vi "Is Call Cancelled.vi"(8 "error in (no error)":errorcluster, 11 "gRPCid in":T1) -> (0 "error out":errorcluster, 2 "Is Cancelled":bool, 3 "gRPCid":T1)   [LabVIEW 2019, in "gprc-lvsupport.lvlib"]
uses:
  gprc-lvsupport.lvlib
  typeDefs/grpcId.ctl
  dlls/labview_grpc_server.dll
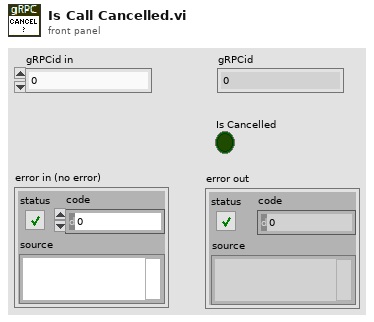
[diagram p1: front panel]
types:
  T1 = typedef "gprc-lvsupport.lvlib/grpcId.ctl" = u64
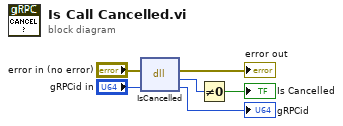
[diagram p0: block diagram]
diagram:
  n1 = dll-call lib="C:/Users/XEnderMD/Desktop/LV gRPC/labview source/gRPC interface/dlls/labview_grpc_server.dll" fn="IsCancelled"(error in="error in (no error)", "id"="gRPCid in") -> (error out=→"error out":errorcluster, "return type"=w4:i32, "id"=→"gRPCid":T1)  [unwired: 2 in, 1 out]
  n2 = Not Equal To 0?(x=w4) -> (x != 0?=→"Is Cancelled":bool)
